vi "SwapInstanceVIUnusedName2 62.vi"(6 "Bindata & descr in":T1, 7 "type":i32, 8 "error in (no error)":errorcluster, 9 "dims":u8=3 min=1 max=3, 11 "kwarg_name":string="testarg") -> (0 "error out":errorcluster, 1 "Array 3D":i32[][][](array[numeric]), 2 "Array 2D":i32[][](array[numeric]), 3 "Array 1D":i32[](array[numeric]), 4 "Bindata & descr out":T1, 5 "bindata":u8[](array[numeric]))   [LabVIEW 2018]
uses:
  Bindata&description.ctl
  Bindata description.ctl
  34ce564e-dc72-4305-b140-1c05df2773d8.vi
  49547b1f-ad21-4c71-9f0b-661b48996dda.vi
  32c0d338-7f1b-4f4e-ba81-eb47dfc88e28.vi
  1cabb67b-d0af-4fb9-bdea-b04621816240.vi
  49547b1f-ad21-4c71-9f0b-661b48996dda.vi/eeead33b-2f9b-414f-8544-d8be5f81d5b2.vi
  32c0d338-7f1b-4f4e-ba81-eb47dfc88e28.vi/36170c27-865a-4dbb-b26a-af3d26789a6c.vi
  1cabb67b-d0af-4fb9-bdea-b04621816240.vi/1332930b-9532-45a3-947e-f1af29da7ac2.vi
  49547b1f-ad21-4c71-9f0b-661b48996dda.vi/eeead33b-2f9b-414f-8544-d8be5f81d5b2.vi/bd9fe851-04a9-4a33-8386-89bfa78ded60.vi
  32c0d338-7f1b-4f4e-ba81-eb47dfc88e28.vi/36170c27-865a-4dbb-b26a-af3d26789a6c.vi/827b2b5a-06d6-478e-9b29-d139325ed30b.vi
  1cabb67b-d0af-4fb9-bdea-b04621816240.vi/1332930b-9532-45a3-947e-f1af29da7ac2.vi/5d77a461-bf35-433b-b13f-ba32f9758be4.vi
  49547b1f-ad21-4c71-9f0b-661b48996dda.vi/eeead33b-2f9b-414f-8544-d8be5f81d5b2.vi/bd9fe851-04a9-4a33-8386-89bfa78ded60.vi/6f90aeee-379a-4374-a4e1-4540642b4bd5.vi
  32c0d338-7f1b-4f4e-ba81-eb47dfc88e28.vi/36170c27-865a-4dbb-b26a-af3d26789a6c.vi/827b2b5a-06d6-478e-9b29-d139325ed30b.vi/a83f1bf5-3cd1-43ae-8b71-873a6c353ca9.vi
  1cabb67b-d0af-4fb9-bdea-b04621816240.vi/1332930b-9532-45a3-947e-f1af29da7ac2.vi/5d77a461-bf35-433b-b13f-ba32f9758be4.vi/c688a18a-f62a-4a25-8c2c-7741d3290a75.vi
  check ID validity.vi
  LV-Julia_ZMQ-Roundtrip_lib.lvlib
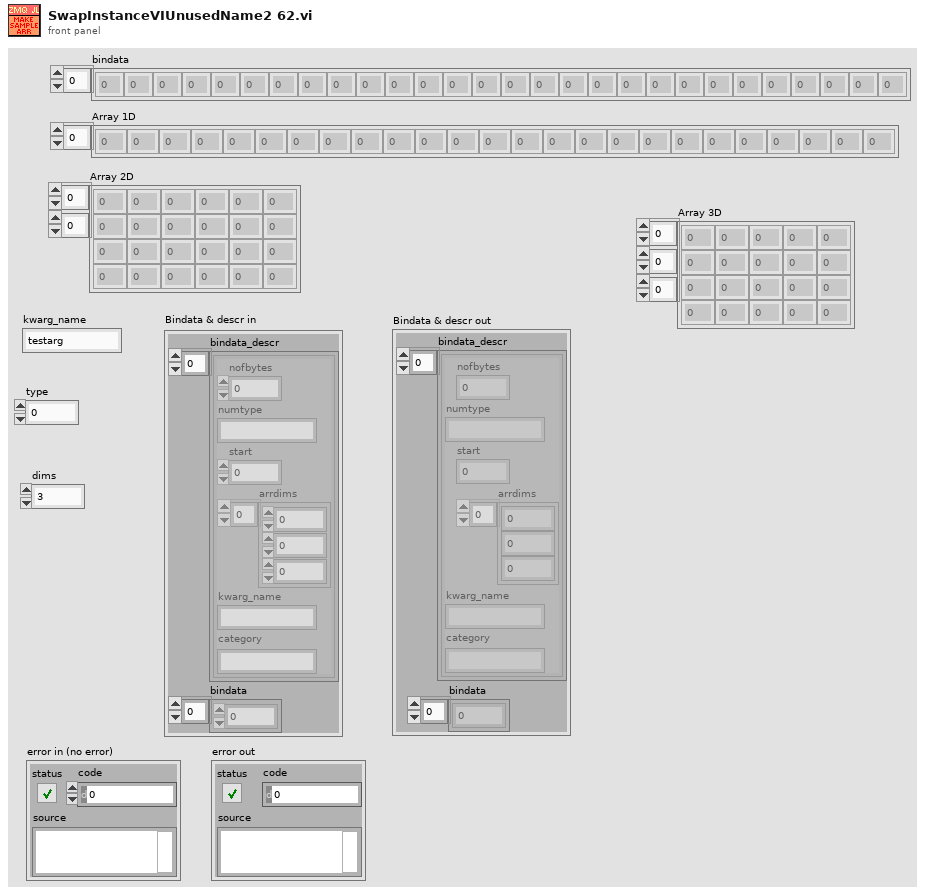
[diagram p1: front panel]
types:
  T1 = typedef "Bindata&description.ctl" = cluster{"bindata_descr":T2[], "bindata":u8[]}
  T2 = typedef "LV-Julia_ZMQ-Roundtrip_lib.lvlib/Bindata description.ctl" = cluster{"nofbytes":i32, "numtype":string, "start":i32, "arrdims":i32[], "kwarg_name":string, "category":string}
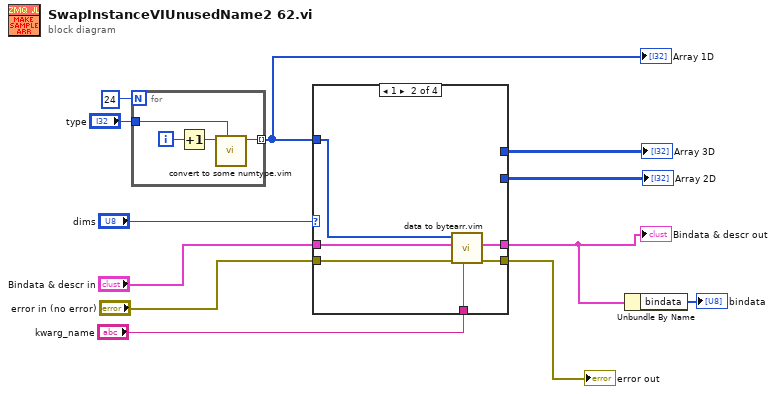
[diagram p0: block diagram]
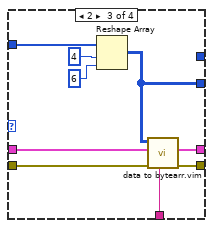
[diagram p3: hidden frame]
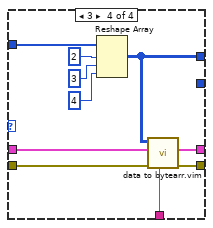
[diagram p4: hidden frame]
diagram:
  n1 = for {
    N: 24 -> [_]
    tunnel: [w14] -> w11 mode=indexing
    tunnel: "type" -> [w13]
    i -> [w16]
    n2 = Increment(x=w16) -> (x+1=w15:i32)
    n3 = call "convert to some numtype.vim"("type"=w13, "Numeric in"=w15) -> ("Numeric out"=w14:i32)  [unwired: 9 in]
  }
  "Array 1D" <- w11
  n4 = case shown="1" "dims" {
    tunnel: [_ _ _ w42] -> w12
    tunnel: w11 -> [_ w23 w30 w38]
    tunnel: "kwarg_name" -> [_ w22 w29 w37]
    tunnel: "error in (no error)" -> [w17 w21 w28 w36]
    tunnel: [w17 w20 w27 w35] -> w5
    tunnel: [_ w19 w26 w34] -> w2
    tunnel: [_ _ w25 _] -> w4
    tunnel: "Bindata & descr in" -> [_ w18 w24 w33]
    frame 0, Default {
    }
    frame 1 {
      n5 = call "data to bytearr.vim"("kwarg_name"=w22, "error in (no error)"=w21, "Bindata & descr in"=w18, "data in"=w23) -> ("error out"=w20:errorcluster, "Bindata & descr out"=w19:T1)  [unwired: 5 in, 1 out]
    }
    frame 2 {
      n6 = Reshape Array(w30, 4 ("dimension size"), 6 ("dimension size")) -> (w25:i32[][])
      n7 = call "data to bytearr.vim"("kwarg_name"=w29, "error in (no error)"=w28, "Bindata & descr in"=w24, "data in"=w25) -> ("error out"=w27:errorcluster, "Bindata & descr out"=w26:T1)  [unwired: 5 in, 1 out]
    }
    frame 3 {
      n8 = Reshape Array(w38, 2 ("dimension size"), 3 ("dimension size"), 4 ("dimension size")) -> (w42:i32[][][])
      n9 = call "data to bytearr.vim"("kwarg_name"=w37, "error in (no error)"=w36, "Bindata & descr in"=w33, "data in"=w42) -> ("error out"=w35:errorcluster, "Bindata & descr out"=w34:T1)  [unwired: 5 in, 1 out]
    }
  }
  "Array 3D" <- w12
  "Bindata & descr out" <- w2
  "error out" <- w5
  "Array 2D" <- w4
  n10 = Unbundle By Name(w2) -> ("bindata"=→"bindata":u8[])
